vi "subDFD_IIR Design.vi"(6 "fs [Hz]":dbl=1.0, 11 "Filter specifications":T7={"Topology"=enum."Butterworth", "Type"=enum."Bandpass", "Order"=6, "Lower Fc"=2000.0, "Upper Fc"=3800.0, "PB Ripple"=0.025, "SB Attenuation"=90.0} {"PB Ripple" format="%0.4f"; "Lower Fc" format="%0.2p"; "SB Attenuation" format="%0.2f"; "Upper Fc" format="%0.2p"}) -> (3 "filter out":T1={"mSRate_Fs"=1.0, "mSRate_Version"="1.0", "mSRate_Comments"="", "mSRate_OrgCoef"={"type"=enum."Undefined", "gain"=1.0, "coef a (k)"=[], "coef b (v)"=[]}, "mSRate_CurCoef"={"type"=enum."Undefined", "gain"=1.0, "coef a (k)"=[], "coef b (v)"=[]}, "mSRate_Quantized?"=FALSE, "mSRate_QCoef"={"type"=enum."Undefined", "gain"=1.0, "coef a (k)"=[], "coef b (v)"=[]}, "mSRate_QSettings"=[], "mSRate_Order"=0, "mSRate_Scaling"={"mSRate_ScaleByPowerOf2?"=FALSE, "mSRate_ScaleType"=enum."No Norm"}} {"mSRate_QSettings"."source" items=["Coef a/k"=0, "Coef b/v"=7, "Input"=1, "Output"=2, "Multiplicand"=3, "Product"=4, "Sum"=5, "Delay"=6, "Gain"=8]})   [LabVIEW 2023]
uses:
  <vilib>/addons/Digital Filter Design/_Objects.llb/DFD Filter Obj.ctl
  <vilib>/addons/Digital Filter Design/_Objects.llb/DFD Filter Coef.ctl
  <vilib>/addons/Digital Filter Design/_Objects.llb/DFD Filter Structure Type Selector.ctl
  <vilib>/addons/Digital Filter Design/_Objects.llb/dfd_Internal Quantization Settings.ctl
  <vilib>/addons/Digital Filter Design/_Objects.llb/dfd_Internal Quantization Srcs.ctl
  <vilib>/addons/Digital Filter Design/_Objects.llb/DFD Coef Norm Type.ctl
  <vilib>/addons/Digital Filter Design/NI_DigFilterLicensed.lvlib
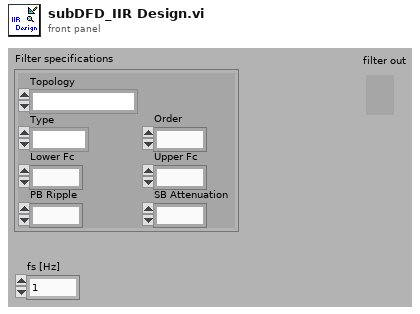
[diagram p1: front panel]
types:
  T1 = typedef "NI_DigFilterLicensed.lvlib/DFD Filter Obj.ctl" = cluster{"mSRate_Fs":dbl, "mSRate_Version":string, "mSRate_Comments":string, "mSRate_OrgCoef":T2, "mSRate_CurCoef":T2, "mSRate_Quantized?":bool, "mSRate_QCoef":T2, "mSRate_QSettings":T4[], "mSRate_Order":i32, "mSRate_Scaling":cluster{"mSRate_ScaleByPowerOf2?":bool, "mSRate_ScaleType":T6}}
  T2 = typedef "NI_DigFilterLicensed.lvlib/DFD Filter Coef.ctl" = cluster{"type":T3, "gain":dbl, "coef a (k)":dbl[], "coef b (v)":dbl[]}
  T3 = typedef "NI_DigFilterLicensed.lvlib/DFD Filter Structure Type Selector.ctl" = enum16{"Undefined", "FIR Direct Form", "FIR Direct Form Transposed", "FIR Symmetric", "FIR Antisymmetric", "IIR Direct Form I", "IIR Direct Form I Transposed", "IIR Direct Form II", "IIR Direct Form II Transposed", "IIR Cascaded Second Order Sections Form I", "IIR Cascaded Second Order Sections Form I Transposed", "IIR Cascaded Second Order Sections Form II", "IIR Cascaded Second Order Sections Form II Transposed", "Lattice Allpass (basic sections)", "Lattice Allpass (one multiplier sections)", "Lattice Allpass (normalized sections)", "Lattice AR (basic sections)", "Lattice AR (one multiplier sections)", "Lattice AR (normalized sections)", "Lattice MA (minimum phase)", "Lattice MA (maximum phase)", "Lattice ARMA (basic sections)", "Lattice ARMA (one multiplier sections)", "Lattice ARMA (normalized sections)"}
  T4 = typedef "NI_DigFilterLicensed.lvlib/dfd_Internal Quantization Settings.ctl" = cluster{"source":T5, "wl":i16, "iwl":i16, "overflow mode":enum16{"Saturation", "Wrap"}, "rounding mode":enum16{"Nearest", "Truncation"}, "signed?":bool}
  T5 = typedef "NI_DigFilterLicensed.lvlib/dfd_Internal Quantization Srcs.ctl" = u16
  T6 = typedef "NI_DigFilterLicensed.lvlib/DFD Coef Norm Type.ctl" = enum16{"No Norm", "Time Domain 1-Norm", "Time Domain 2-Norm", "Time Domain Inf-Norm"}
  T7 = cluster{"Topology":enum16{"Off", "Butterworth", "Chebyshev", "Inverse Chebyshev", "Elliptic", "Bessel"}, "Type":enum16{"Lowpass", "Highpass", "Bandpass", "Bandstop"}, "Order":i32, "Lower Fc":dbl, "Upper Fc":dbl, "PB Ripple":dbl, "SB Attenuation":dbl}
  T8 = enum16{"Lowpass", "Highpass", "Bandpass", "Bandstop"}
  T9 = enum16{"Off", "Butterworth", "Chebyshev", "Inverse Chebyshev", "Elliptic", "Bessel"}
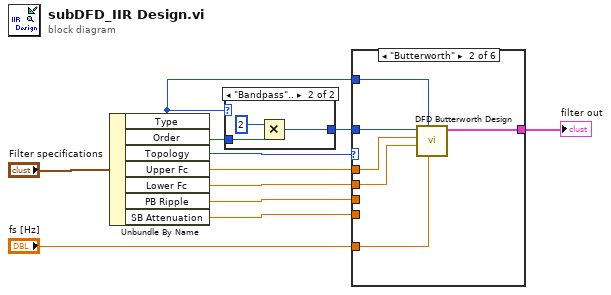
[diagram p0: block diagram]
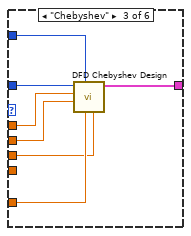
[diagram p4: hidden frame]
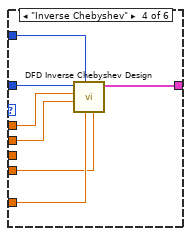
[diagram p5: hidden frame]
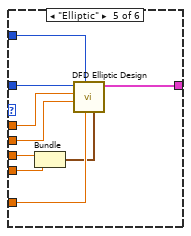
[diagram p6: hidden frame]
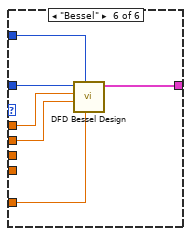
[diagram p7: hidden frame]
diagram:
  n1 = Unbundle By Name("Filter specifications") -> ("Type"=w3:T8, "Order"=w5:i32, "Topology"=w6:T9, "Upper Fc"=w10:dbl, "Lower Fc"=w9:dbl, "PB Ripple"=w8:dbl, "SB Attenuation"=w7:dbl)
  n2 = case shown="\"Bandpass\".." w3 {
    tunnel: w5 -> [w12 w15]
    tunnel: [w12 w13] -> w4
    frame "Lowpass", Default {
    }
    frame "Bandpass".. {
      n3 = Multiply(x=2, y=w15) -> (x*y=w13:i32)
    }
  }
  n4 = case shown="\"Butterworth\"" w6 {
    tunnel: w10 -> [_ w19 w26 w33 w42 w48]
    tunnel: w9 -> [_ w18 w25 w32 w41 w47]
    tunnel: w8 -> [_ _ w22 _ w38 _]
    tunnel: w7 -> [_ _ _ w29 w37 _]
    tunnel: w4 -> [_ w21 w28 w35 w44 w50]
    tunnel: w3 -> [_ w20 w27 w34 w43 w49]
    tunnel: "fs [Hz]" -> [_ w17 w24 w31 w40 w46]
    tunnel: [_ w16 w23 w30 w39 w45] -> w1
    frame "Off", Default {
    }
    frame "Butterworth" {
      n5 = call <vilib>:"DFD Butterworth Design.vi"("fs [Hz]"=w17, "filter type"=w20, "low cutoff freq [Hz]"=w18, "high cutoff freq [Hz]"=w19, "order"=w21) -> ("filter out"=w16:T1)  [unwired: 1 in, 5 out]
    }
    frame "Chebyshev" {
      n6 = call <vilib>:"DFD Chebyshev Design.vi"("passband ripple [dB]"=w22, "fs [Hz]"=w24, "filter type"=w27, "low cutoff freq [Hz]"=w25, "high cutoff freq [Hz]"=w26, "order"=w28) -> ("filter out"=w23:T1)  [unwired: 1 in, 4 out]
    }
    frame "Inverse Chebyshev" {
      n7 = call <vilib>:"DFD Inverse Chebyshev Design.vi"("stopband atten [dB]"=w29, "fs [Hz]"=w31, "filter type"=w34, "low cutoff freq [Hz]"=w32, "high cutoff freq [Hz]"=w33, "order"=w35) -> ("filter out"=w30:T1)  [unwired: 1 in, 4 out]
    }
    frame "Elliptic" {
      n8 = Bundle("PB Ripple"=w38, "SB Attenuation"=w37) -> (w36:cluster{"PB Ripple":dbl, "SB Attenuation":dbl})  [unwired: 1 out]
      n9 = call <vilib>:"DFD Elliptic Design.vi"("ripples [dB]"=w36, "fs [Hz]"=w40, "filter type"=w43, "low cutoff freq [Hz]"=w41, "high cutoff freq [Hz]"=w42, "order"=w44) -> ("filter out"=w39:T1)  [unwired: 1 in, 4 out]
    }
    frame "Bessel" {
      n10 = call <vilib>:"DFD Bessel Design.vi"("fs [Hz]"=w46, "filter type"=w49, "low cutoff freq [Hz]"=w47, "high cutoff freq [Hz]"=w48, "order"=w50) -> ("filter out"=w45:T1)  [unwired: 2 in, 4 out]
    }
  }
  "filter out" <- w1
